vi "8matrici_led.vi"() -> ()   [LabVIEW 2018]
panel:
  out "Temp":u32
  in  "Meter":u32(knob) scale=0.0..10.0
  in  "stop":bool
  out "Matrice 8":bool[][](array[boolean])
  out "Matrice 7":bool[][](array[boolean])
  out "Matrice 6":bool[][](array[boolean])
  out "Matrice 5":bool[][](array[boolean])
  out "Matrice 4":bool[][](array[boolean])
  out "Matrice 3":bool[][](array[boolean])
  out "Matrice 2":bool[][](array[boolean])
  in  "Start":bool
  in  "cadru":string(combo)
  out "Matrice 1":bool[][](array[boolean])
  in  "Main":bool[][](array[boolean])
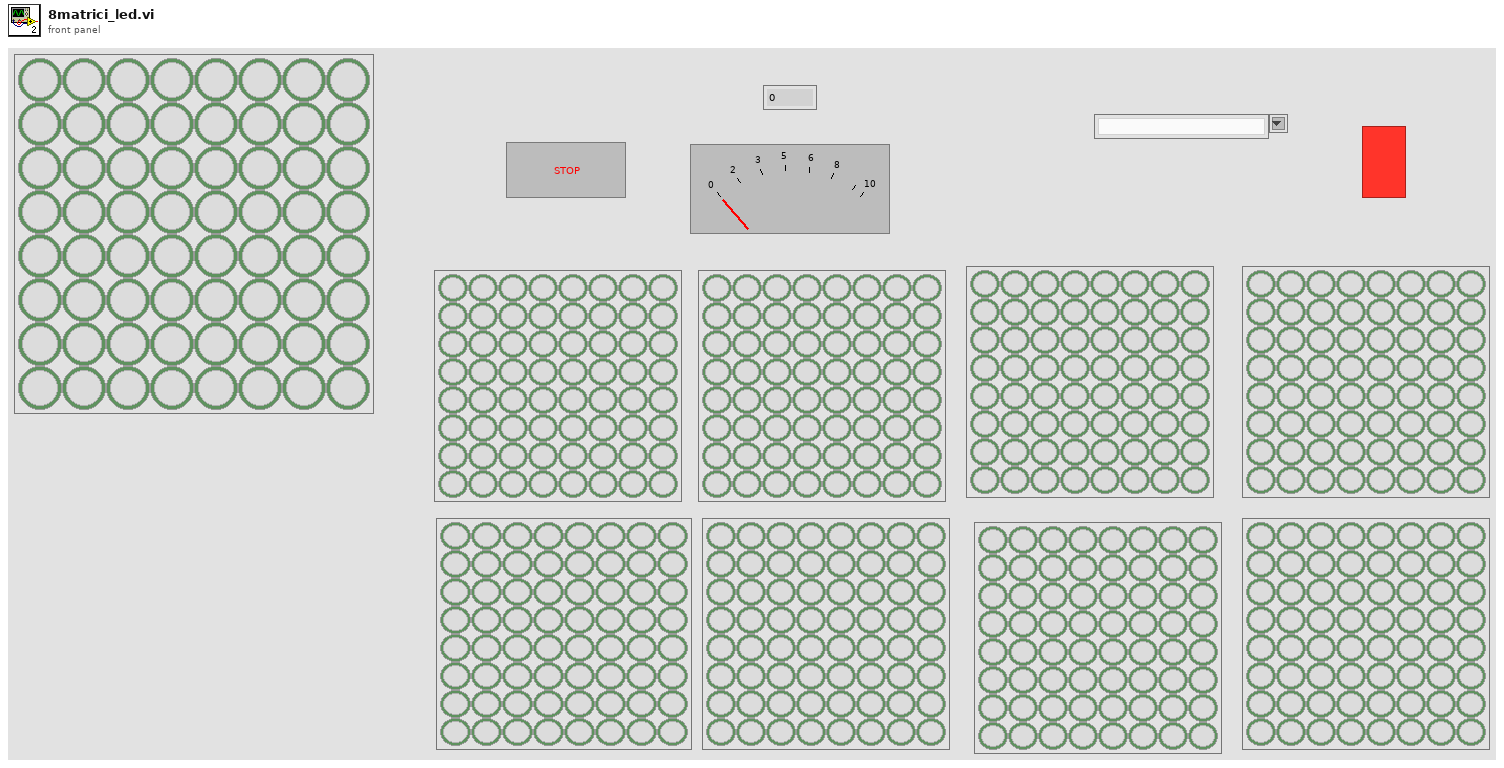
[diagram p1: front panel]
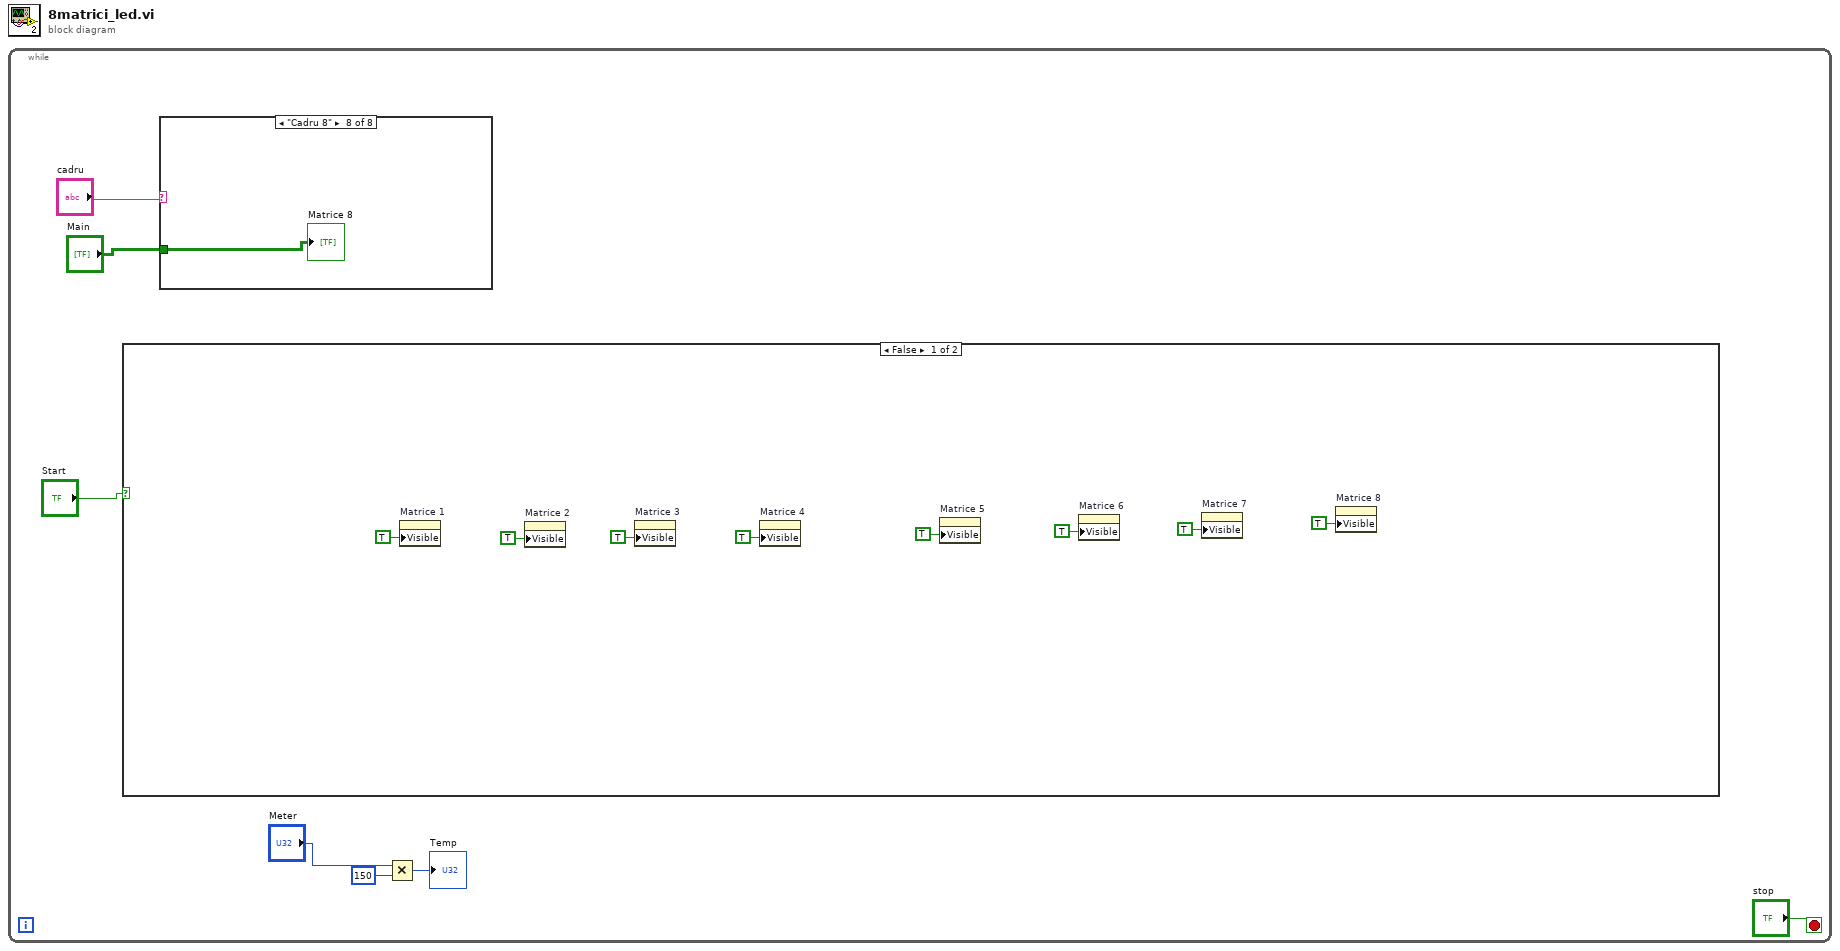
[diagram p0: block diagram]
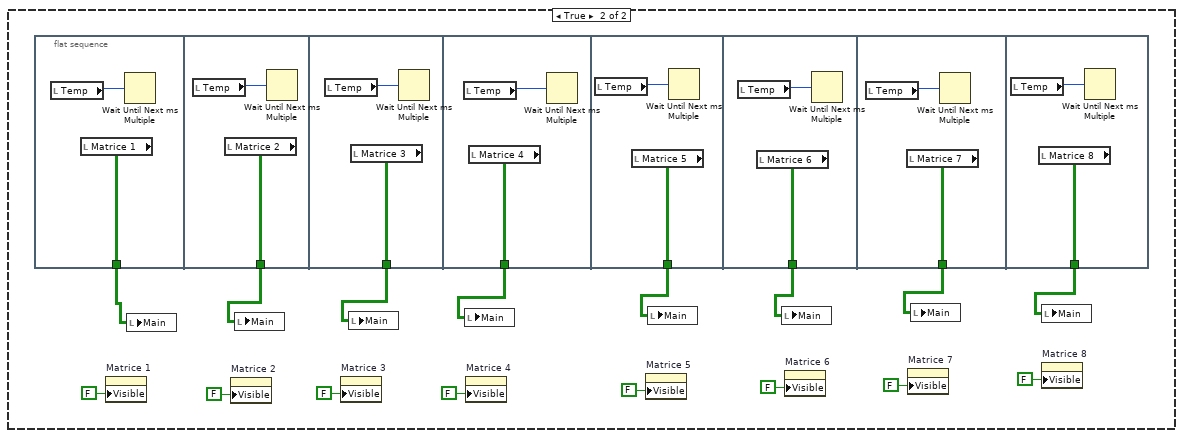
[diagram p2: hidden frame]
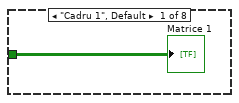
[diagram p3: hidden frame]
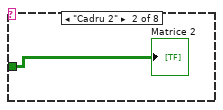
[diagram p4: hidden frame]
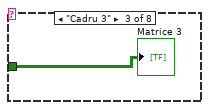
[diagram p5: hidden frame]
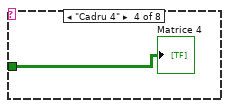
[diagram p6: hidden frame]
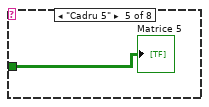
[diagram p7: hidden frame]
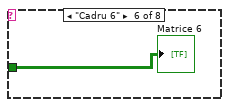
[diagram p8: hidden frame]
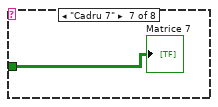
[diagram p9: hidden frame]
diagram:
  n1 = while {
    stop <- "stop" stop-if-true
    n2 = case shown="False" "Start" {
      frame False {
        n3 = property on="Matrice 1" class="Arr (strict)"("Visible"=TRUE) -> ()  [unwired: 2 in, 2 out]
        n4 = property on="Matrice 2" class="Arr (strict)"("Visible"=TRUE) -> ()  [unwired: 2 in, 2 out]
        n5 = property on="Matrice 3" class="Arr (strict)"("Visible"=TRUE) -> ()  [unwired: 2 in, 2 out]
        n6 = property on="Matrice 4" class="Arr (strict)"("Visible"=TRUE) -> ()  [unwired: 2 in, 2 out]
        n7 = property on="Matrice 5" class="Arr (strict)"("Visible"=TRUE) -> ()  [unwired: 2 in, 2 out]
        n8 = property on="Matrice 6" class="Arr (strict)"("Visible"=TRUE) -> ()  [unwired: 2 in, 2 out]
        n9 = property on="Matrice 7" class="Arr (strict)"("Visible"=TRUE) -> ()  [unwired: 2 in, 2 out]
        n10 = property on="Matrice 8" class="Arr (strict)"("Visible"=TRUE) -> ()  [unwired: 2 in, 2 out]
      }
      frame True {
        n11 = flat-sequence {
          tunnel: [w33] -> w24
          tunnel: [w35] -> w25
          tunnel: [w37] -> w26
          tunnel: [w39] -> w27
          tunnel: [w41] -> w28
          tunnel: [w43] -> w29
          tunnel: [w45] -> w30
          tunnel: [w47] -> w31
          frame #0 {
            n12 = local read "Temp"() -> (w32:u32)
            n13 = local read "Matrice 1"() -> (w33:bool[][])
            n14 = Wait Until Next ms Multiple(millisecond multiple=w32) -> ()  [unwired: 1 out]
          }
          frame #1 {
            n15 = local read "Temp"() -> (w34:u32)
            n16 = local read "Matrice 2"() -> (w35:bool[][])
            n17 = Wait Until Next ms Multiple(millisecond multiple=w34) -> ()  [unwired: 1 out]
          }
          frame #2 {
            n18 = local read "Temp"() -> (w36:u32)
            n19 = local read "Matrice 3"() -> (w37:bool[][])
            n20 = Wait Until Next ms Multiple(millisecond multiple=w36) -> ()  [unwired: 1 out]
          }
          frame #3 {
            n21 = local read "Temp"() -> (w38:u32)
            n22 = local read "Matrice 4"() -> (w39:bool[][])
            n23 = Wait Until Next ms Multiple(millisecond multiple=w38) -> ()  [unwired: 1 out]
          }
          frame #4 {
            n24 = local read "Temp"() -> (w40:u32)
            n25 = local read "Matrice 5"() -> (w41:bool[][])
            n26 = Wait Until Next ms Multiple(millisecond multiple=w40) -> ()  [unwired: 1 out]
          }
          frame #5 {
            n27 = local read "Temp"() -> (w42:u32)
            n28 = local read "Matrice 6"() -> (w43:bool[][])
            n29 = Wait Until Next ms Multiple(millisecond multiple=w42) -> ()  [unwired: 1 out]
          }
          frame #6 {
            n30 = local read "Temp"() -> (w44:u32)
            n31 = local read "Matrice 7"() -> (w45:bool[][])
            n32 = Wait Until Next ms Multiple(millisecond multiple=w44) -> ()  [unwired: 1 out]
          }
          frame #7 {
            n33 = local read "Temp"() -> (w46:u32)
            n34 = local read "Matrice 8"() -> (w47:bool[][])
            n35 = Wait Until Next ms Multiple(millisecond multiple=w46) -> ()  [unwired: 1 out]
          }
        }
        n36 = property on="Matrice 1" class="Arr (strict)"("Visible"=FALSE) -> ()  [unwired: 2 in, 2 out]
        n37 = local write "Main"(w24) -> ()
        n38 = property on="Matrice 2" class="Arr (strict)"("Visible"=FALSE) -> ()  [unwired: 2 in, 2 out]
        n39 = local write "Main"(w25) -> ()
        n40 = property on="Matrice 3" class="Arr (strict)"("Visible"=FALSE) -> ()  [unwired: 2 in, 2 out]
        n41 = local write "Main"(w26) -> ()
        n42 = local write "Main"(w27) -> ()
        n43 = property on="Matrice 4" class="Arr (strict)"("Visible"=FALSE) -> ()  [unwired: 2 in, 2 out]
        n44 = property on="Matrice 5" class="Arr (strict)"("Visible"=FALSE) -> ()  [unwired: 2 in, 2 out]
        n45 = local write "Main"(w28) -> ()
        n46 = local write "Main"(w29) -> ()
        n47 = property on="Matrice 6" class="Arr (strict)"("Visible"=FALSE) -> ()  [unwired: 2 in, 2 out]
        n48 = property on="Matrice 7" class="Arr (strict)"("Visible"=FALSE) -> ()  [unwired: 2 in, 2 out]
        n49 = local write "Main"(w30) -> ()
        n50 = local write "Main"(w31) -> ()
        n51 = property on="Matrice 8" class="Arr (strict)"("Visible"=FALSE) -> ()  [unwired: 2 in, 2 out]
      }
    }
    n52 = case shown="\"Cadru 8\"" "cadru" {
      tunnel: "Main" -> [w48 w49 w50 w51 w52 w53 w54 w55]
      frame "Cadru 1", Default {
        "Matrice 1" <- w48
      }
      frame "Cadru 2" {
        "Matrice 2" <- w49
      }
      frame "Cadru 3" {
        "Matrice 3" <- w50
      }
      frame "Cadru 4" {
        "Matrice 4" <- w51
      }
      frame "Cadru 5" {
        "Matrice 5" <- w52
      }
      frame "Cadru 6" {
        "Matrice 6" <- w53
      }
      frame "Cadru 7" {
        "Matrice 7" <- w54
      }
      frame "Cadru 8" {
        "Matrice 8" <- w55
      }
    }
    n53 = Multiply(x="Meter", y=u32 150) -> (x*y=→"Temp":u32)
  }
